vi "badgeuse.vi"(1 "VISA resource name":refnum<visa-resource-name> caption="Nom de ressource VISA") -> (0 "sous-chaîne correspondante":string)   [LabVIEW 2024]
uses:
  <vilib>/drjdpowell/SQLite Library/SQL Connection/Open (string).vi
  <vilib>/Utility/error.llb/Trim Whitespace One-Sided.vi
  <vilib>/Instr/_visa.llb/VISA Configure Serial Port (Instr).vi
  <vilib>/drjdpowell/SQLite Library/SQL Connection/Execute SQL (No results).vi
  <vilib>/drjdpowell/SQLite Library/SQL Connection/Connection.lvclass
  <vilib>/drjdpowell/SQLite Library/SQLite.lvlib
panel:
  out "offset après correspondance":i32
  out "buffer de lecture":string
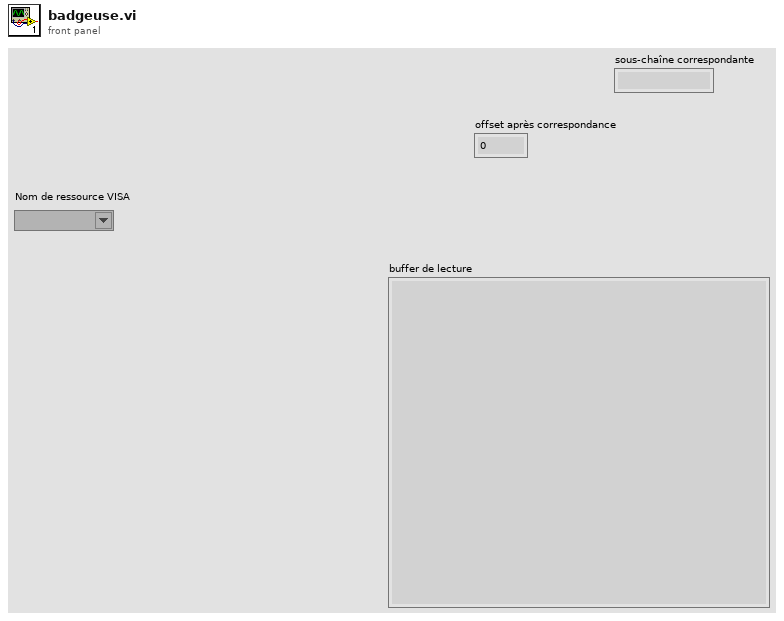
[diagram p1: front panel]
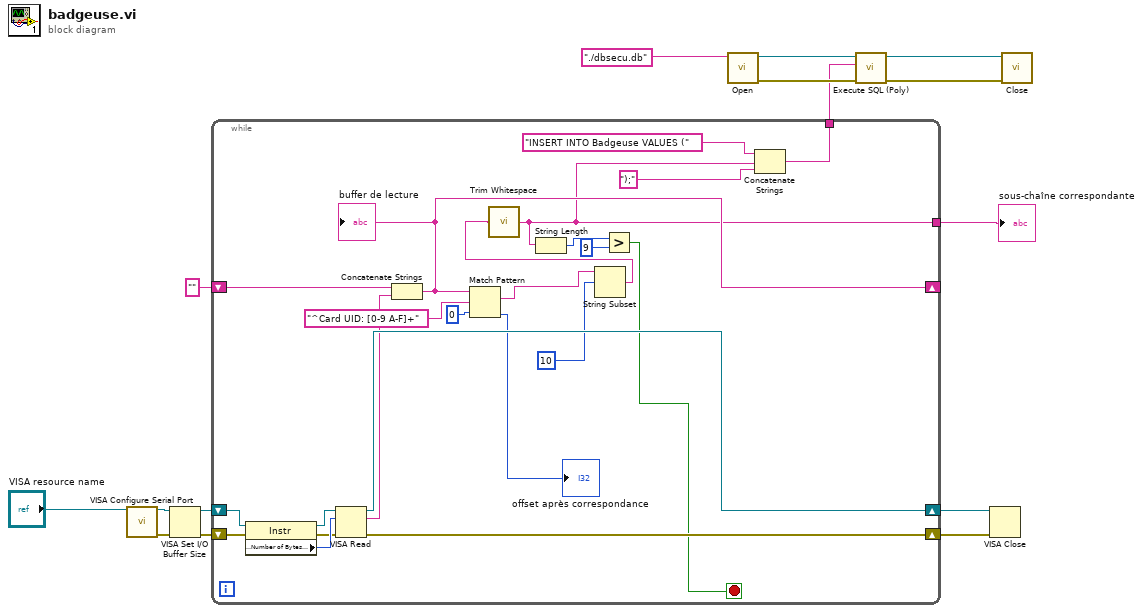
[diagram p0: block diagram]
diagram:
  n1 = call-poly "VISA Configure Serial Port"("VISA resource name"="VISA resource name") -> ("VISA resource name out"=w15:refnum<visa-resource-name>, "error out"=w14:errorcluster)  [unwired: 13 in]
  n2 = VISA Set I/O Buffer Size(VISA resource name=w15, error in (no error)=w14) -> (VISA resource name out=w12:refnum<visa-resource-name>, error out=w13:errorcluster)  [unwired: 2 in]
  n3 = while {
    shift-right: [w37] -> w10
    shift-left: w12 -> [w31]
    shift-right: [w38] -> w11
    shift-left: w13 -> [w33]
    shift-right: [w27] -> _
    shift-left: "" -> [w36]
    tunnel: [w18] -> w6
    tunnel: [w16] -> w1
    stop <- w20 stop-if-true
    n4 = property class="Instr"(reference=w31, error in=w33) -> (reference out=w30:refnum<visa-resource-name>, error out=w32:errorcluster, "Serial Settings:Number of Bytes at Serial Port"=w34:u32)
    n5 = VISA Read(VISA resource name=w30, byte count=w34, error in (no error)=w32) -> (VISA resource name out=w37:refnum<visa-resource-name>, read buffer=w35:string, error out=w38:errorcluster)  [unwired: 1 out]
    n6 = Concatenate Strings(w36, w35) -> (w27:string)
    "buffer de lecture" <- w27
    n7 = Match Pattern(string=w27, regular expression="^Card UID: [0-9 A-F]+" ("expression régulière"), offset (0)=0) -> (match substring=w25:string, offset past match=→"offset après correspondance":i32)  [unwired: 2 out]
    n8 = String Subset(string=w25, offset (0)=10) -> (substring=w23:string)  [unwired: 1 in]
    n9 = call <vilib>:"Trim Whitespace.vi"("string"=w23) -> ("trimmed string"=w18:string)  [unwired: 1 in]
    n10 = String Length(string=w18) -> (length=w22:i32)
    n11 = Greater?(x=w22, y=9) -> (0:w20:bool)
    n12 = Concatenate Strings("INSERT INTO Badgeuse VALUES (", w18, ");") -> (w16:string)
  }
  "sous-chaîne correspondante" <- w6
  n13 = call-poly <vilib>:"Open.vi"("db file"="./dbsecu.db") -> ("error out"=w5:errorcluster, "SQLite Connection"=w4:refnum<class "Connection.lvclass">)  [unwired: 9 in]
  n14 = call-poly <vilib>:"Execute SQL (Poly).vi"("error in (no error)"=w5, "SQL"=w1, "SQLite Connection in"=w4) -> ("error out"=w3:errorcluster, "SQLite Connection"=w2:refnum<class "Connection.lvclass">)  [unwired: 7 in]
  n15 = VISA Close(VISA resource name=w10, error in (no error)=w11) -> ()  [unwired: 1 out]
  n16 = call-dynamic "Close.vi"("error in (no error)"=w3, "SQLite Connection in"=w2) -> ()  [unwired: 9 in, 1 out]
